vi "UDPrecieverMin2Bin.vi"() -> ()   [LabVIEW 2012]
panel:
  out "substring":string
  out "error post-check":errorcluster
  out "End Reciever Error":errorcluster
  in  "stop reciever":bool
  out "port":u16
  out "error out post-read":errorcluster
  out "error out pre-read":errorcluster
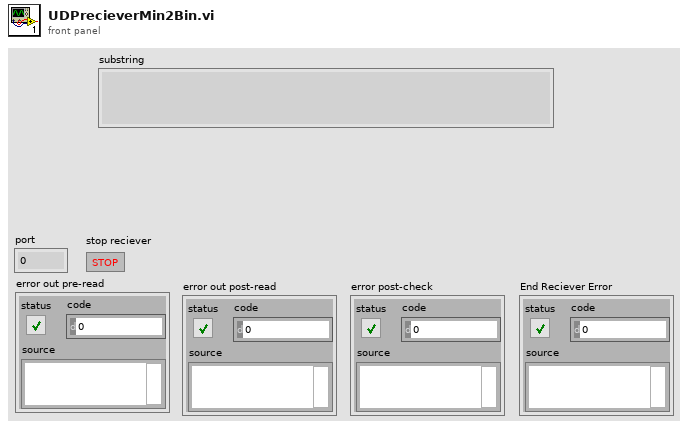
[diagram p1: front panel]
types:
  T1 = enum16{"open", "replace", "create", "open or create", "replace or create", "replace or create with confirmation"}
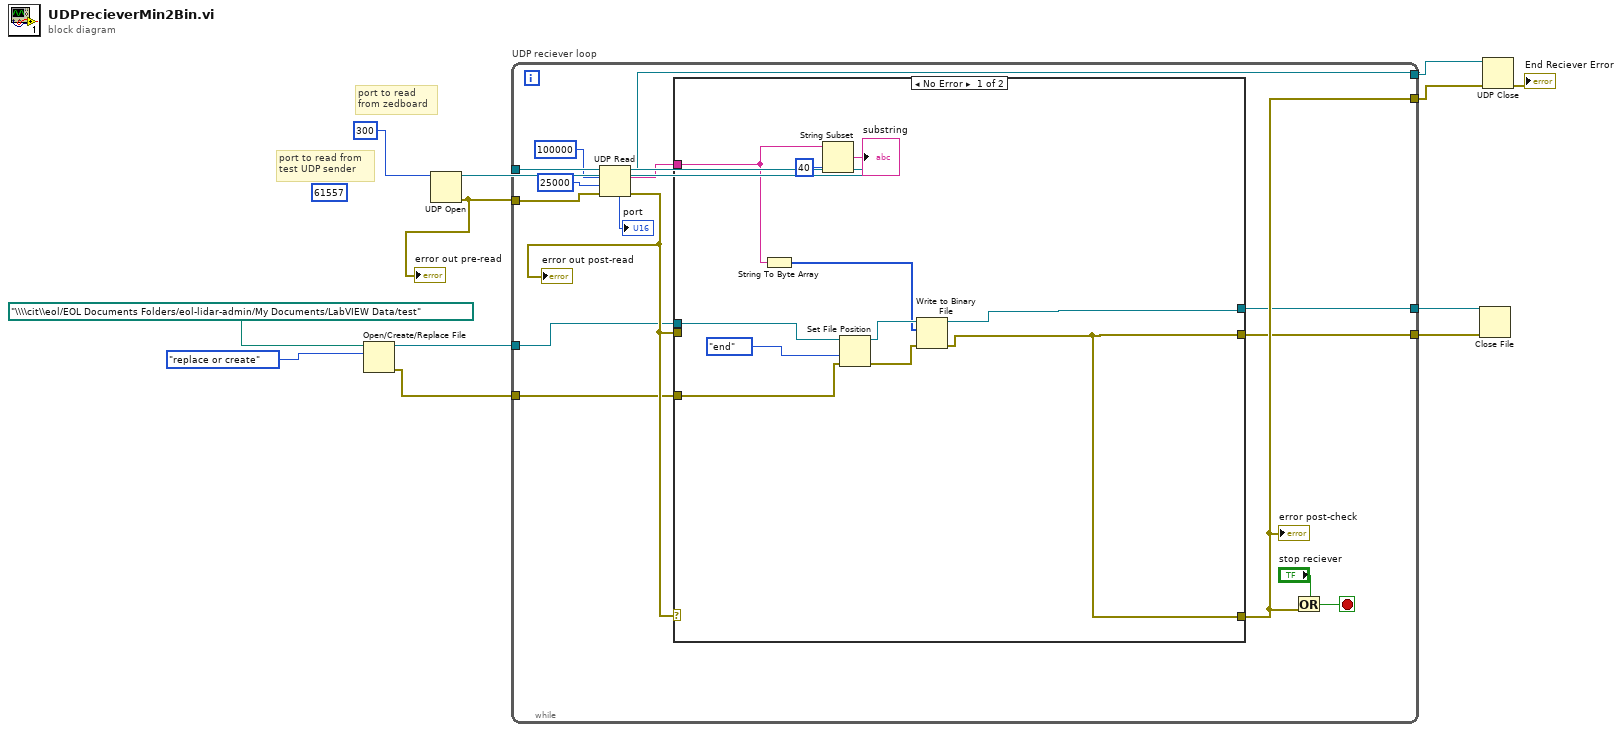
[diagram p0: block diagram]
diagram:
  (unwired) u16 61557 ("port")
  # "port to read \nfrom zedboard"
  # "port to read from \ntest UDP sender"
  n1 = Open/Create/Replace File(file path (use dialog)=path "\\\\cit\\eol/EOL Documents Folders/eol-lidar-admin/My Documents/LabVIEW Data/test" ("file (use dialog)"), operation (0:open)=T1."replace or create") -> (refnum out=w5:refnum<file>, error out=w3:errorcluster)  [unwired: 4 in, 1 out]
  n2 = UDP Open(11:u16 300 ("port")) -> (port=w11:refnum<k16>, 0:w8:errorcluster)  [unwired: 4 in, 1 out]
  "error out pre-read" <- w8
  n3 = while "UDP reciever loop" {
    tunnel: [w27] -> w12
    tunnel: w11 -> [w26]
    tunnel: [w19] -> w10
    tunnel: w8 -> [w23]
    tunnel: w5 -> [w16]
    tunnel: w3 -> [w15]
    tunnel: [w14] -> w2
    tunnel: [w13] -> w1
    stop <- w25 stop-if-true
    n4 = UDP Read(connection ID=w26, max size (548)=100000, timeout ms (25000)=25000, 8:w23) -> (data out=w21:string, error out=w17:errorcluster, 3:w27:refnum<k16>, 4:→"port":u16)  [unwired: 1 out]
    "error out post-read" <- w17
    n5 = case shown="No Error" w17 {
      selector: w17 -> [_ w41]
      tunnel: w21 -> [w30 _]
      tunnel: [w32 w41] -> w19
      tunnel: w17 -> [_ _]
      tunnel: w16 -> [w37 w40]
      tunnel: w15 -> [w36 w39]
      tunnel: [w32 w39] -> w14
      tunnel: [w31 w40] -> w13
      frame No Error {
        n6 = String To Byte Array(string=w30) -> (unsigned byte array=w33:u8[])
        n7 = String Subset(string=w30, length (rest)=40 ("length (rest)")) -> (substring=→"substring":string)  [unwired: 1 in]
        n8 = Set File Position(refnum=w37, from (0:start)=enum16{"start", "end", "current"}."end", error in=w36) -> (refnum out=w34:refnum<file>, error out=w35:errorcluster)  [unwired: 1 in]
        n9 = Write to Binary File(file (use dialog)=w34, data=w33, error in=w35) -> (refnum out=w31:refnum<file>, error out=w32:errorcluster)  [unwired: 3 in, 1 out]
      }
      frame Error {
      }
    }
    "error post-check" <- w19
    n10 = Or(x="stop reciever", y=w19) -> (x .or. y?=w25:bool)
  }
  n11 = Close File(refnum=w1, error in=w2) -> ()  [unwired: 2 out]
  n12 = UDP Close(connection ID=w12, 8:w10) -> (error out=→"End Reciever Error":errorcluster)  [unwired: 1 out]
